vi "LV6_2.vi"() -> ()   [LabVIEW 2011]
uses:
  <vilib>/sound2/lvsound2.llb/Sampling Mode.ctl
  <vilib>/Utility/file.llb/Read From Spreadsheet File (DBL).vi
  <vilib>/imath/engines/lvmath2/RunTimeEngine/ErrorHandling/NIMS_Finalize Error.vi
  <vilib>/imath/engines/lvmath2/RunTimeEngine/BuiltInFunctions/length/NIMS_length(GV).vi
  <instcachedir>/0/NIMS_length(GV)_08A3D13377FD4E4B96F5795FBF3698FA.lvgen/NIMS_length(GV)_08A3D13377FD4E4B96F5795FBF3698FA_000.vi
  <vilib>/imath/engines/lvmath2/RunTimeEngine/NodeEndStatement/NIMS_NodeEndStatement_Output.vi
  <instcachedir>/0/NIMS_NodeEndStatement_Output_53EC0D466D134D7ABD903AC30B43404B.lvgen/NIMS_NodeEndStatement_Output_53EC0D466D134D7ABD903AC30B43404B_002.vi
  <instcachedir>/0/NIMS_NodeEndStatement_Output_53EC0D466D134D7ABD903AC30B43404B.lvgen/NIMS_NodeEndStatement_Output_53EC0D466D134D7ABD903AC30B43404B_005.vi
  <instcachedir>/0/NIMS_NodeEndStatement_Output_53EC0D466D134D7ABD903AC30B43404B.lvgen/NIMS_NodeEndStatement_Output_53EC0D466D134D7ABD903AC30B43404B_009.vi
  <vilib>/imath/engines/lvmath2/RunTimeEngine/RangeToken/NIMS_Range.vi
  <instcachedir>/0/NIMS_Range_0B7635FB69F84E19AA68E7FF959DF37C.lvgen/NIMS_Range_0B7635FB69F84E19AA68E7FF959DF37C_000.vi
  <vilib>/imathl/engines/lvmath/Functions/Error Handling/Create Error.vi
  <vilib>/imath/engines/lvmath2/RunTimeEngine/BuiltInFunctions/poly/NIMS_GV=poly(GV).vi
  <instcachedir>/0/NIMS_GV=poly(GV)_A1C8B7C92C4F409DB664B03EC1C81090.lvgen/NIMS_GV=poly(GV)_A1C8B7C92C4F409DB664B03EC1C81090_000.vi
  <vilib>/imath/engines/lvmath2/RunTimeEngine/ErrorHandling/NIMS_Create Error From Enums.vi
  <vilib>/imath/engines/lvmath2/RunTimeEngine/BuiltInFunctions/residue/NIMS_residue_To Partial Fraction Expansion.vi
  <vilib>/imath/engines/lvmath2/RunTimeEngine/ErrorHandling/NIMS_Error From Error Code.vi
  <vilib>/imath/engines/lvmath2/RunTimeEngine/ArithmeticOperatorToken/NIMS_ArithmeticOperator_multmx.vi
  <instcachedir>/0/NIMS_ArithmeticOperator_multmx_7C179C1E3F6A47AEB223A71AB1A54D0B.lvgen/NIMS_ArithmeticOperator_multmx_7C179C1E3F6A47AEB223A71AB1A54D0B_006.vi
  <vilib>/imath/engines/lvmath2/RunTimeEngine/ArithmeticOperatorToken/NIMS_ArithmeticOperator_multmx(RV,M).vi
  <instcachedir>/0/NIMS_ArithmeticOperator_multmx(RV,M)_0F69384DF375434AAFCFC7849B80E797.lvgen/NIMS_ArithmeticOperator_multmx(RV,M)_0F69384DF375434AAFCFC7849B80E797_000.vi
  <vilib>/imath/engines/lvmath2/RunTimeEngine/BuiltInFunctions/fft/NIMS_fft(GM).vi
  <instcachedir>/0/NIMS_fft(GM)_4927013A90BC44B4B38EF4F7AFCEDB88.lvgen/NIMS_fft(GM)_4927013A90BC44B4B38EF4F7AFCEDB88_000.vi
  <vilib>/imath/engines/lvmath2/RunTimeEngine/BuiltInFunctions/fft/NIMS_fft(GV).vi
  <instcachedir>/0/NIMS_fft(GV)_4C6467FC22F84E4BA42517A07EF978B0.lvgen/NIMS_fft(GV)_4C6467FC22F84E4BA42517A07EF978B0_000.vi
  <vilib>/imath/engines/lvmath2/RunTimeEngine/ArithmeticOperatorToken/NIMS_ArithmeticOperator_times.vi
  <instcachedir>/0/NIMS_ArithmeticOperator_times_3FA9DDB491BD45F6905798C0465C9825.lvgen/NIMS_ArithmeticOperator_times_3FA9DDB491BD45F6905798C0465C9825_001.vi
  <vilib>/imath/engines/lvmath2/RunTimeEngine/BuiltInFunctions/ifft/NIMS_ifft(CM).vi
  <vilib>/imath/engines/lvmath2/RunTimeEngine/ArithmeticOperatorToken/NIMS_ArithmeticOperator_plus.vi
  <instcachedir>/0/NIMS_ArithmeticOperator_plus_1E95F7DAB906458CBECCADBE8E6FD739.lvgen/NIMS_ArithmeticOperator_plus_1E95F7DAB906458CBECCADBE8E6FD739_003.vi
  <vilib>/imath/engines/lvmath2/RunTimeEngine/VariableToken/Read/NIMS_Get Elements - SorM(_) - Check.vi
  <instcachedir>/0/NIMS_Get Elements - SorM(_) - Check_6C920A4996D9400D8D9F035318A663F0.lvgen/NIMS_Get Elements - SorM(_) - Check_6C920A4996D9400D8D9F035318A663F0_007.vi
  <vilib>/imath/engines/lvmath2/RunTimeEngine/BuiltInFunctions/abs/NIMS_abs(signed).vi
  <instcachedir>/0/NIMS_abs(signed)_C4FCB8E6058B49B797C7C8D53CA5F6EC.lvgen/NIMS_abs(signed)_C4FCB8E6058B49B797C7C8D53CA5F6EC_003.vi
  <vilib>/imath/engines/lvmath2/RunTimeEngine/VariableToken/Read/NIMS_Get Elements - RV(_) - Check.vi
  <instcachedir>/0/NIMS_Get Elements - RV(_) - Check_B511B9D8E05044FE80F9F088FE24B20C.lvgen/NIMS_Get Elements - RV(_) - Check_B511B9D8E05044FE80F9F088FE24B20C_003.vi
  <instcachedir>/0/NIMS_abs(signed)_C4FCB8E6058B49B797C7C8D53CA5F6EC.lvgen/NIMS_abs(signed)_C4FCB8E6058B49B797C7C8D53CA5F6EC_006.vi
  <vilib>/sound2/lvsound2.llb/Sound Output Write (DBL Single).vi
panel:
  in  "order":i32(slide)=9 scale=2.0..10.0
  out "Filter  (frequency domain)":cluster{"F":dbl[], "FYI":dbl[]}(graph)
  in  "minus real part of poles":dbl(slide)=100.0 scale=10.0..100.0
  in  "fundamental frequency":dbl(slide)=435.0 scale=300.0..500.0
  out "Filter impulse (time domain)":cluster{"t":dbl[], "Y":dbl[]}(graph)
  out "Filtered (frequency domain)":cluster{"F":dbl[], "FYI":dbl[]}(graph)
  out "Original signal (frequency domain)":cluster{"F":dbl[], "FXI":dbl[]}(graph)
  out "Original signal (time domain)":cluster{"t":dbl[], "first row":dbl[]}(graph)
  out "Filtered signal (time domain)":cluster{"t":dbl[], "Y":dbl[]}(graph)
  in  "Play original sound":bool
  in  "Play filtered sound":bool
  in  "stop":bool
  # "A note = 440 Hz"
  # "G note = 392 Hz"
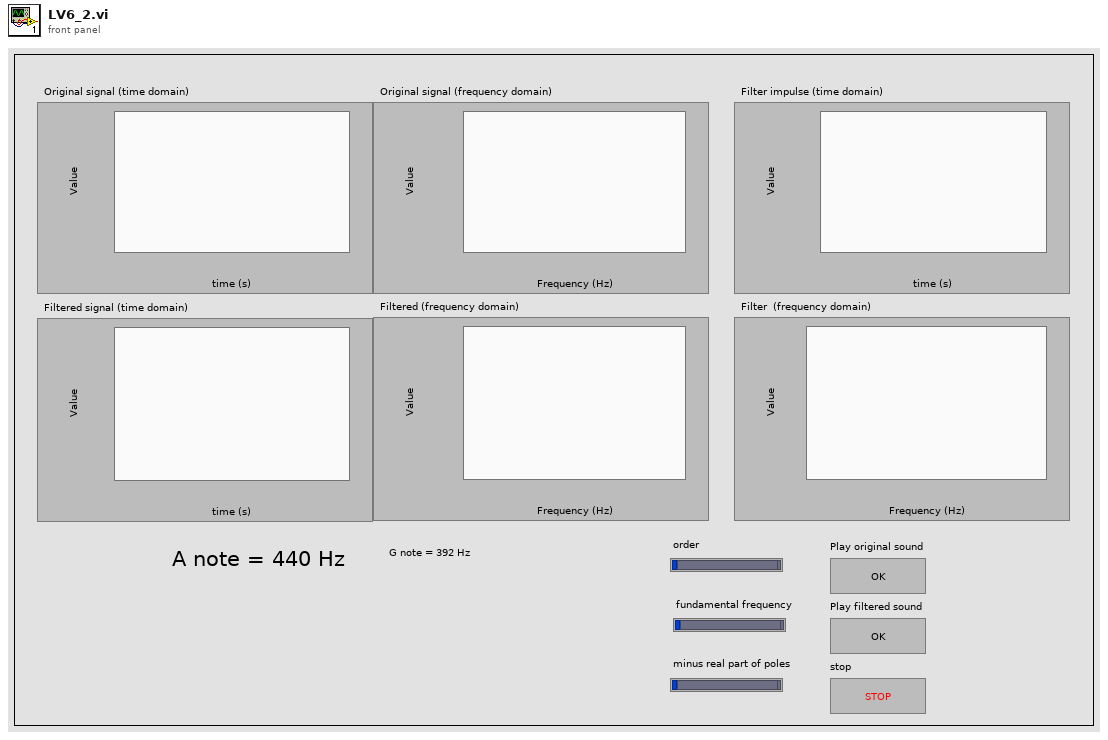
[diagram p1: front panel]
types:
  T1 = typedef "Sampling Mode.ctl" = i32
  T2 = typedef "Sound Output Task ID.ctl" = u32
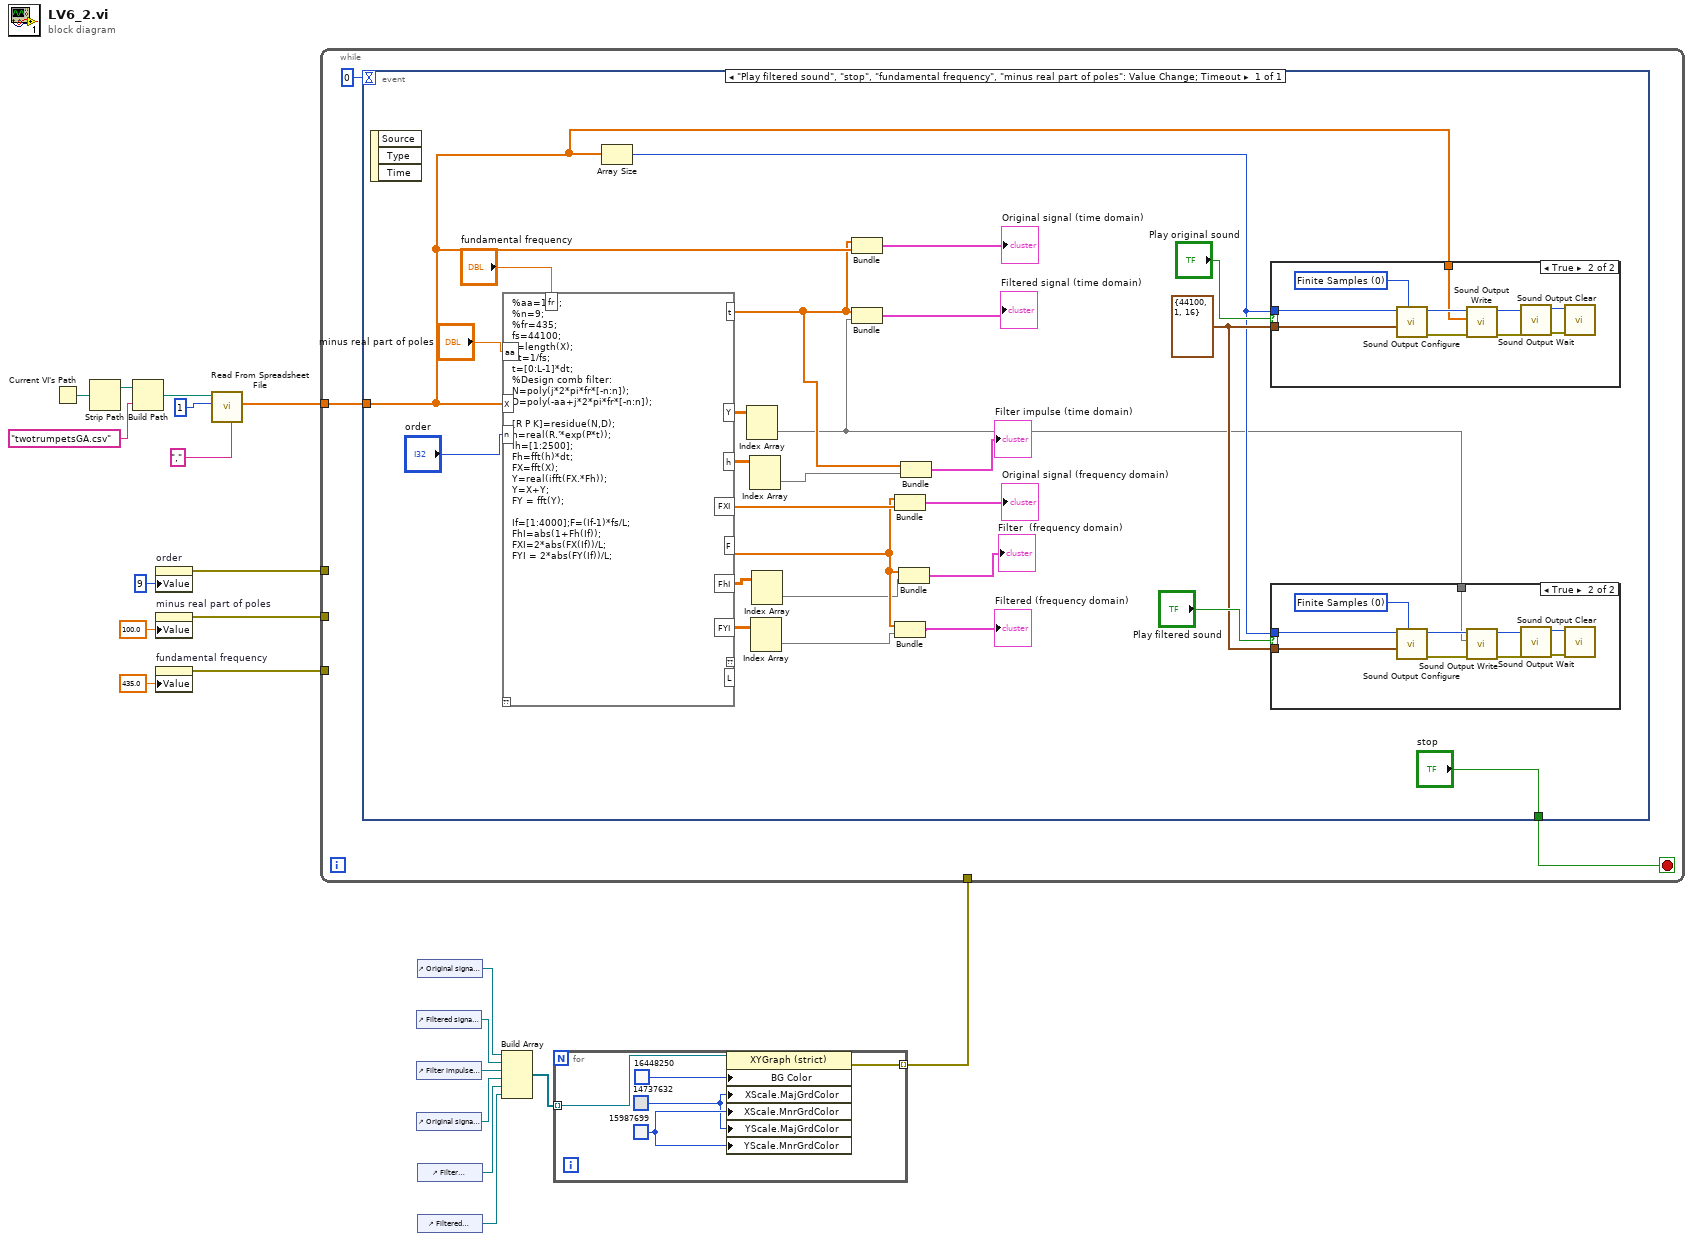
[diagram p0: block diagram]
diagram:
  n1 = Current VI's Path() -> (path=w21:path)
  n2 = Strip Path(path=w21) -> (stripped path=w20:path)  [unwired: 1 out]
  n3 = Build Path(base path=w20, name or relative path="twotrumpetsGA.csv") -> (appended path=w18:path)
  n4 = property on="order" class="Slide (strict)"("Value"=9 ("order")) -> (error out=w14:errorcluster)  [unwired: 2 in, 1 out]
  n5 = property on="minus real part of poles" class="Slide (strict)"("Value"=100.0 ("minus real part of poles")) -> (error out=w13:errorcluster)  [unwired: 2 in, 1 out]
  n6 = property on="fundamental frequency" class="Slide (strict)"("Value"=435.0 ("fundamental frequency")) -> (error out=w12:errorcluster)  [unwired: 2 in, 1 out]
  n7 = call-poly <vilib>:"Read From Spreadsheet File.vi"("delimiter (\\t)"="," ("delimiter (\\t)"), "number of rows (all:-1)"=1, "file path (dialog if empty)"=w18) -> ("first row"=w15:dbl[])  [unwired: 4 in, 4 out]
  n8 = control-ref of="Filtered signal (time domain)"() -> (w6:refnum<vi>)
  n9 = control-ref of="Filter impulse (time domain)"() -> (w5:refnum<vi>)
  n10 = control-ref of="Original signal (frequency domain)"() -> (w4:refnum<vi>)
  n11 = control-ref of="Original signal (time domain)"() -> (w7:refnum<vi>)
  n12 = control-ref of="Filter  (frequency domain)"() -> (w3:refnum<vi>)
  n13 = control-ref of="Filtered (frequency domain)"() -> (w2:refnum<vi>)
  n14 = Build Array(w7, w6, w5, w4, w3, w2) -> (w8:refnum<vi>[])
  n15 = for {
    tunnel: w8 -> [w22] mode=indexing
    tunnel: [w23] -> w1 mode=indexing
    w25 = u32 15987699
    w24 = u32 14737632
    n16 = property class="XYGraph (strict)"(reference=w22, "BG Color"=u32 16448250, "XScale.MajGrdColor"=w24, "XScale.MnrGrdColor"=w25, "YScale.MajGrdColor"=w24, "YScale.MnrGrdColor"=w25) -> (error out=w23:errorcluster)  [unwired: 1 in, 1 out]
  }
  n17 = while {
    tunnel: w15 -> [w29]
    tunnel: w14 -> [_]
    tunnel: w13 -> [_]
    tunnel: w12 -> [_]
    tunnel: w1 -> [_]
    stop <- w28 stop-if-true
    n18 = event shown="[0] \"Play filtered sound\", \"stop\", \"fundamental frequency\", \"minus real part of poles\": Value Change;  Timeout" {
      selector: _ -> [_]
      dyn-events: _ -> [_]
      timeout: 0 -> [_]
      tunnel: w29 -> [w52]
      tunnel: ["stop"] -> w28
      event "Play filtered sound", "stop", "fundamental frequency", "minus real part of poles": Value Change; Timeout {
        w50 = cluster{"fs":i32, i32, i32} {"fs"=44100, 1, 16}
        n19 = event-data() -> ()  [unwired: 1 in, 3 out]
        n20 = mathscript code="%aa=100;\n%n=9;\n%fr=435;\nfs=44100;\nL=length(X);\ndt=1/fs;\nt=[0:L-1]*dt;\n%Design comb filter:\nN=poly(j*2*pi*fr*[-n:n]);\nD=poly(-aa+j*2*pi*fr*[-n:n]);\n\n[R P K]=residue(N,D);\nh=real(R.'*exp(P*t));\nIh=[1:2500];\nFh=fft(h)*dt;\nFX=fft(X);\nY=real(ifft(FX.*Fh));\nY=X+Y;\nFY = fft(Y);\n\nIf=[1:4000];F=(If-1)*fs/L;\nFhI=abs(1+Fh(If));\nFXI=2*abs(FX(If))/L;\nFYI = 2*abs(FY(If))/L;"("X"=w52, "aa"="minus real part of poles", "fr"="fundamental frequency", "n"="order") -> ("Y"=w42:dbl[][], "F"=w46:dbl[], "FYI"=w35:dbl[][], "t"=w43:dbl[], "FXI"=w47:dbl[], "FhI"=w37:dbl[][], "h"=w40:dbl[][])  [unwired: 1 in, 2 out]
        n21 = Array Size(array=w52) -> (size(s)=w49:i32)
        n22 = Index Array(array=w42) -> (element=w41:dbl[])  [unwired: 2 in]
        n23 = Index Array(array=w40) -> (element=w39:dbl[])  [unwired: 2 in]
        n24 = Index Array(array=w35) -> (element=w34:dbl[])  [unwired: 2 in]
        n25 = Index Array(array=w37) -> (element=w36:dbl[])  [unwired: 2 in]
        n26 = Bundle("t"=w43, "first row"=w52) -> (→"Original signal (time domain)":cluster{"t":dbl[], "first row":dbl[]})  [unwired: 1 in]
        n27 = Bundle("t"=w43, "Y"=w41) -> (→"Filtered signal (time domain)":cluster{"t":dbl[], "Y":dbl[]})  [unwired: 1 in]
        n28 = Bundle("F"=w46, "FXI"=w47) -> (→"Original signal (frequency domain)":cluster{"F":dbl[], "FXI":dbl[]})  [unwired: 1 in]
        n29 = Bundle("F"=w46, "FYI"=w34) -> (→"Filtered (frequency domain)":cluster{"F":dbl[], "FYI":dbl[]})  [unwired: 1 in]
        n30 = Bundle("F"=w46, "FhI"=w36) -> (→"Filter  (frequency domain)":cluster{"F":dbl[], "FhI":dbl[]})  [unwired: 1 in]
        n31 = Bundle("t"=w43, "h"=w39) -> (→"Filter impulse (time domain)":cluster{"t":dbl[], "h":dbl[]})  [unwired: 1 in]
        n32 = case shown="True" "Play original sound" {
          tunnel: w50 -> [_ w364]
          tunnel: w49 -> [_ w362]
          tunnel: w52 -> [_ w361]
          frame False {
          }
          frame True {
            w363 = T1 0 items=["Finite Samples", "Continuous Samples"] ("sample mode")
            n33 = call <vilib>:"Sound Output Configure.vi"("number of samples/ch"=w362, "sample mode"=w363, "sound format"=w364) -> ("error out"=w365:errorcluster, "task ID"=w370:T2)  [unwired: 7 in]
            n34 = call-poly <vilib>:"Sound Output Write.vi"("error in (no error)"=w365, "data"=w361, "task ID"=w370) -> ("error out"=w366:errorcluster, "task ID out"=w367:T2)  [unwired: 7 in]
            n35 = call <vilib>:"Sound Output Wait.vi"("error in (no error)"=w366, "task ID"=w367) -> ("error out"=w369:errorcluster, "task ID out"=w368:T2)  [unwired: 8 in]
            n36 = call <vilib>:"Sound Output Clear.vi"("error in (no error)"=w369, "task ID"=w368) -> ()  [unwired: 9 in, 1 out]
          }
        }
        n37 = case shown="True" "Play filtered sound" {
          tunnel: w50 -> [_ w354]
          tunnel: w49 -> [_ w352]
          tunnel: w41 -> [_ w351]
          frame False {
          }
          frame True {
            w353 = T1 0 items=["Finite Samples", "Continuous Samples"] ("sample mode")
            n38 = call <vilib>:"Sound Output Configure.vi"("number of samples/ch"=w352, "sample mode"=w353, "sound format"=w354) -> ("error out"=w355:errorcluster, "task ID"=w360:T2)  [unwired: 7 in]
            n39 = call-poly <vilib>:"Sound Output Write.vi"("error in (no error)"=w355, "data"=w351, "task ID"=w360) -> ("error out"=w356:errorcluster, "task ID out"=w357:T2)  [unwired: 7 in]
            n40 = call <vilib>:"Sound Output Wait.vi"("error in (no error)"=w356, "task ID"=w357) -> ("error out"=w359:errorcluster, "task ID out"=w358:T2)  [unwired: 8 in]
            n41 = call <vilib>:"Sound Output Clear.vi"("error in (no error)"=w359, "task ID"=w358) -> ()  [unwired: 9 in, 1 out]
          }
        }
      }
    }
  }
